vi "Get Value.vi"(8 "error in (no error)":errorcluster, 11 "PathTreeNode in":refnum<class "PathTreeNode.lvclass">) -> (0 "error out":errorcluster, 2 "Value":refnum<class>, 3 "PathTreeNode out":refnum<class "PathTreeNode.lvclass">)   [LabVIEW 2020, in "Advanced Structures.lvlib" / "PathTreeNode.lvclass"]
uses:
  PathTreeNode.lvclass
  PathTreeNode.lvclass/PathTreeNode.ctl
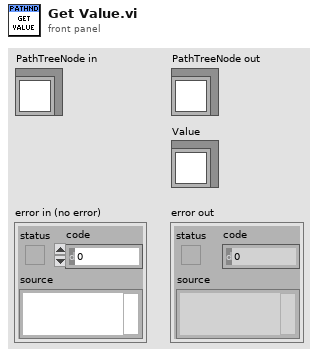
[diagram p1: front panel]
types:
  T1 = typedef "Advanced Structures.lvlib/PathTreeNode.lvclass/Ref Data.ctl" = cluster{"Tree":refnum<class>, "Parent":refnum<class>, "Token":string, "Child Tokens":string[], "Child Nodes":refnum<class>[], "Value":refnum<class>, "Has Value":bool}
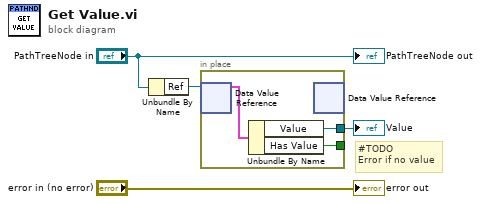
[diagram p0: block diagram]
diagram:
  # "#TODO\nError if no value"
  n1 = Unbundle By Name("PathTreeNode in") -> ("Ref"=w3:refnum<data-value>)
  n2 = in-place {
    in-place-border: [w6] -> w1
    in-place-border: [w5] -> _
    n3 = in-place-dvr #1(w3) -> (w7:T1)  [unwired: 1 out]
    n4 = Unbundle By Name(w7) -> ("Value"=w6:refnum<class>, "Has Value"=w5:bool)
    n5 = in-place-dvr #1() -> ()  [unwired: 1 in, 2 out]
  }
  "Value" <- w1
  "error out" <- "error in (no error)"
  "PathTreeNode out" <- "PathTreeNode in"
